vi "Radar-Vital-Sign.vi"() -> ()   [LabVIEW 2014]
doc: "Personal Daq 54 example.\nTriggering is immediate and readings are returned 1 scan at a time as available.\nBe sure to use the Acquisition Stop control for proper shutdown."
uses:
  <vilib>/Utility/error.llb/DialogType.ctl
  <vilib>/DAQmx/read.llb/DAQmx Read (Analog 1D DBL NChan 1Samp).vi
  <vilib>/Analysis/2dsp.llb/Complex FFT.vi
  <vilib>/DAQmx/create/channels.llb/DAQmx Create Channel (AI-Voltage-Basic).vi
  <vilib>/DAQmx/configure/timing.llb/DAQmx Timing (Sample Clock).vi
  <vilib>/DAQmx/miscellaneous.llb/DAQmx Fill In Error Info.vi
  <vilib>/measure/madcrms.llb/Basic Averaged DC-RMS for 1 Chan.vi
  Instance           2 26Saved   noise_Nov07_2009_5 .vi
  Instance          18 26Saved   noise_Nov07_2009_5 .vi
  Instance           4 26Saved   noise_Nov07_2009_5 .vi
  Instance           1 26Saved   noise_Nov07_2009_5 .vi
  <vilib>/measure/NI_MAPro.lvlib
  <vilib>/Analysis/NI_AALPro.lvlib
panel:
  in  "Save Data":bool
  in  "Max. Heartrate":i32=90
  in  "Min. Heartrate":i32=50
  out "Heartrate":dbl
  in  "Max. Resp. Rate":i32=30
  in  "Min. Resp. Rate":i32=10
  out "Resp. Rate":dbl
  in  "input terminal configuration":i32(ring)=10083 items=["default"=-1, "RSE"=10083, "NRSE"=10078, "Differential"=10106, "Pseudodifferential"=12529]
  in  "stop":bool
  in  "Maximum Value":dbl=5.0 format="%0.2f"
  in  "Minimum Value":dbl=-2.0 format="%0.2f"
  in  "Rate":dbl=20.0 caption="Sample Rate (Hz)" format="%0.2f"
  in  "Samples per Channel":i32=1
  out "Combined Spectrum":waveform(dbl)(graph)
  in  "FFT":i32=256
  out "I/Q Signal":dynamicdata(graph)
  in  "t0":timestamp=timestamp(3198752888.296 s since 1904-01-01)
  # "Radar Noncontact Vital Sign Detection\n\nby C.Gu, April 2012\n@ Texas Tech"
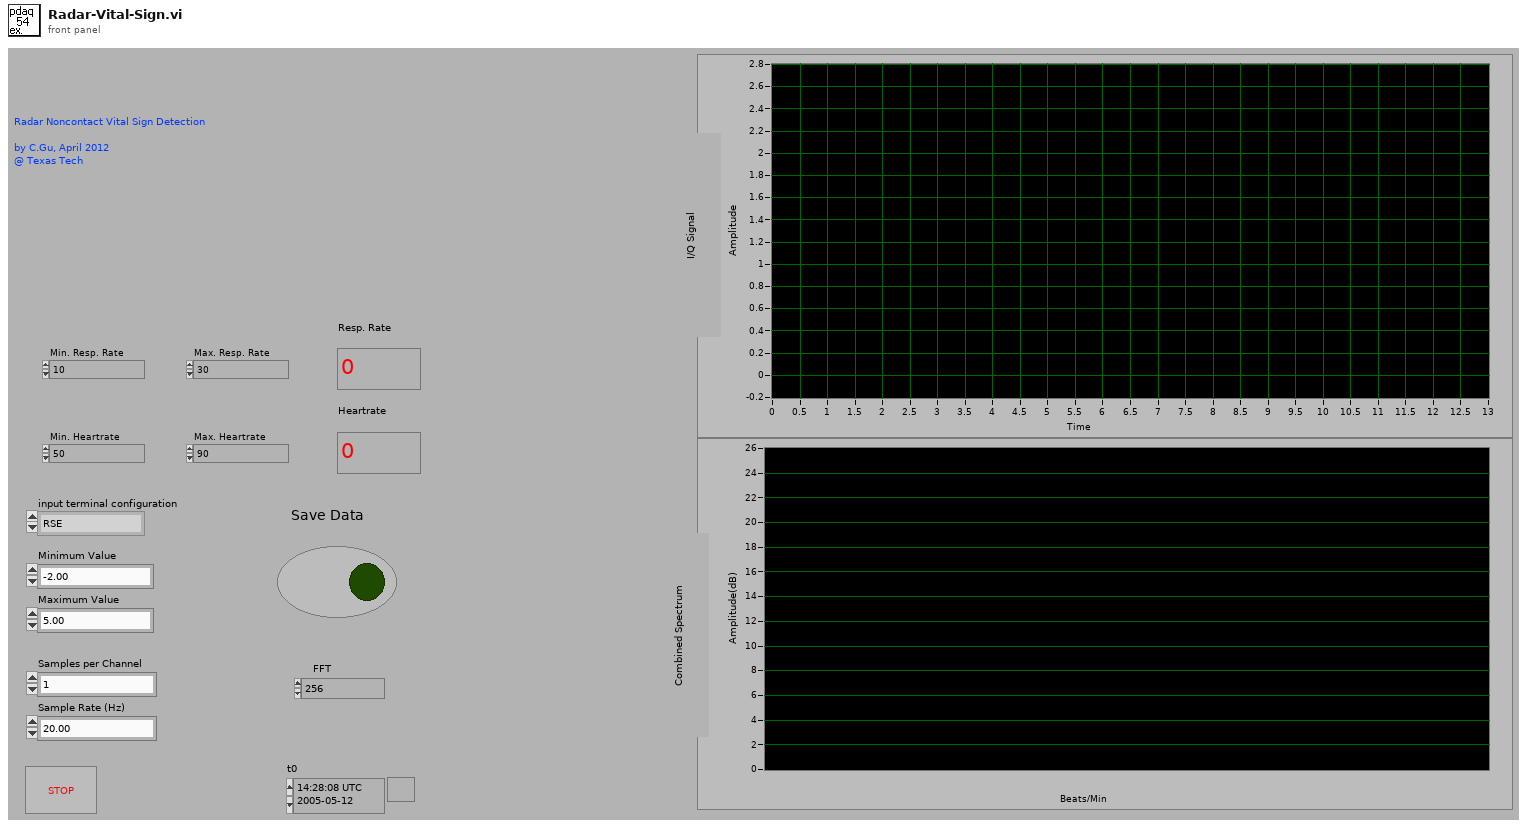
[diagram p1: front panel]
types:
  T1 = typedef "DialogType.ctl" = u16
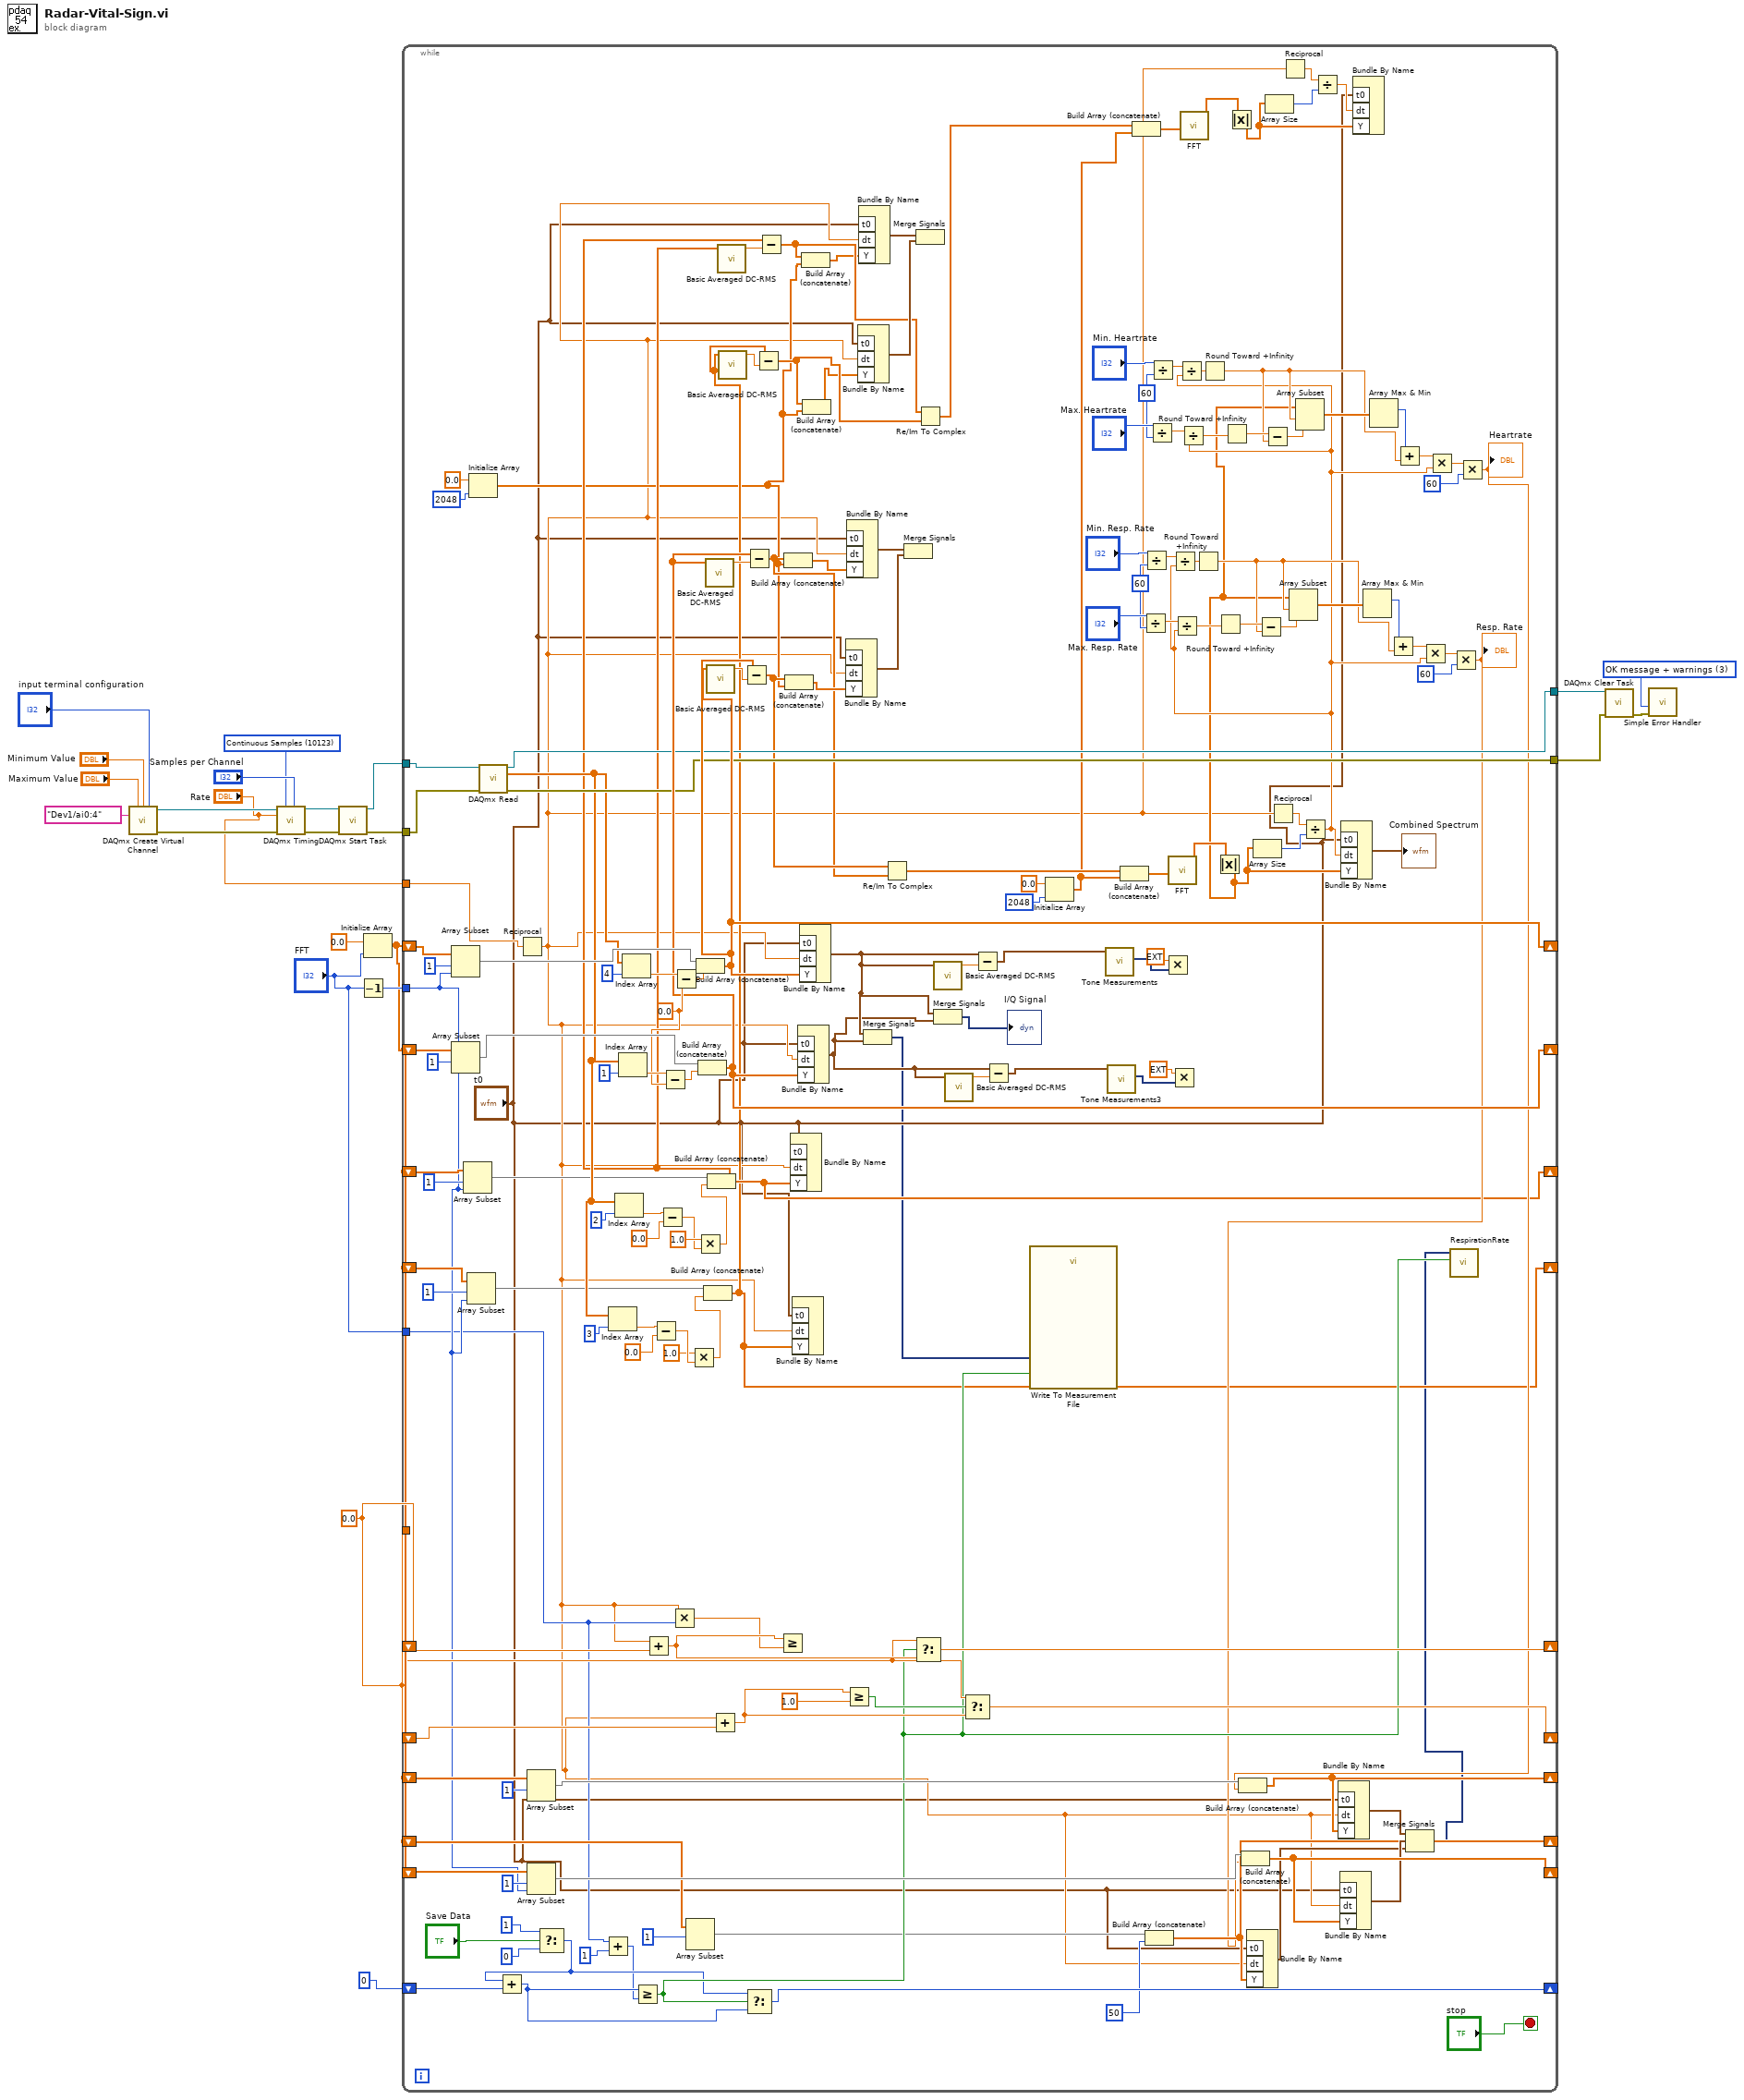
[diagram p0: block diagram]
diagram:
  w3 = 0.0 ("element")
  w9 = T1 3 items=["no dialog", "OK message", "continue or stop message", "OK message + warnings", "continue/stop + warnings"] ("type of dialog (OK msg:1)")
  w16 = 10123 items=["Finite Samples"=10178, "Continuous Samples"=10123] ("sample mode")
  n1 = call-poly <vilib>:"DAQmx Create Virtual Channel.vi"("maximum value"="Maximum Value", "minimum value"="Minimum Value", "input terminal configuration"="input terminal configuration", "physical channels"=tag "Dev1/ai0:4") -> ("task out"=w17:refnum<k21>, "error out"=w19:errorcluster)  [unwired: 5 in, 5 out]
  n2 = call-poly <vilib>:"DAQmx Timing.vi"("task/channels in"=w17, "sample mode"=w16, "samples per channel"="Samples per Channel", "rate"="Rate", "error in"=w19) -> ("task out"=w15:refnum<k21>, "error out"=w14:errorcluster)  [unwired: 2 in, 7 out]
  n3 = call <vilib>:"DAQmx Start Task.vi"("task/channels in"=w15, "error in"=w14) -> ("task out"=w12:refnum<k21>, "error out"=w11:errorcluster)  [unwired: 12 out]
  n4 = Decrement(x="FFT") -> (x-1=w22:i32)
  n5 = Initialize Array(0.0 ("element"), "FFT") -> (w1:dbl[])
  n6 = while {
    shift-right: [w156] -> _
    shift-left: w1 -> [w186]
    tunnel: w22 -> [w62]
    shift-right: [w155] -> _
    shift-left: w1 -> [w177]
    tunnel: w12 -> [w154]
    tunnel: w11 -> [w153]
    tunnel: "Rate" -> [w152]
    tunnel: [w151] -> w8
    tunnel: [w150] -> w7
    shift-right: [w145] -> _
    shift-left: w3 -> [w143]
    tunnel: "FFT" -> [w51]
    tunnel: w3 -> [w137]
    shift-right: [w141] -> _
    shift-left: w3 -> [w138]
    shift-right: [w125] -> _
    shift-left: w1 -> [w131]
    shift-right: [w126] -> _
    shift-left: w1 -> [w128]
    shift-right: [w86] -> _
    shift-left: 0 -> [w88]
    shift-right: [w44] -> _
    shift-left: w1 -> [w79]
    shift-right: [w70] -> _
    shift-left: w1 -> [w74]
    shift-right: [w43] -> _
    shift-left: w1 -> [w64]
    stop <- "stop" stop-if-true
    w91 = 60
    w106 = 60
    w171 = 0.0 ("element")
    n7 = Array Subset(array=w186, index=1, length=w62) -> (w184:dbl[])
    n8 = Array Subset(array=w177, index=1, length=w62) -> (w175:dbl[])
    n9 = Array Subset(array=w79, index=1, length=w62) -> (w45:dbl[])
    n10 = Array Subset(array=w64, index=1, length=w62) -> (w54:dbl[])
    n11 = Initialize Array(0.0 ("element"), 2048 ("dimension size")) -> (w40:dbl[])
    n12 = call-poly <vilib>:"DAQmx Read.vi"("task/channels in"=w154, "error in"=w153) -> ("task out"=w151:refnum<k21>, "data"=w55:dbl[], "error out"=w150:errorcluster)  [unwired: 11 out]
    n13 = Reciprocal(x=w152) -> (1/x=w29:dbl)
    n14 = Array Subset(array=w128, index=1) -> (w127:dbl[])  [unwired: 1 in]
    n15 = Array Subset(array=w131, index=1, length=w62) -> (w130:dbl[])
    n16 = Select(t=1, s="Save Data", f=0) -> (s? t:f=w82:i32)
    n17 = Add(x=w82, y=w88) -> (x+y=w87:i32)
    n18 = Add(x=w51, y=1 ("index")) -> (x+y=w50:i32)
    n19 = Index Array(array=w55, index=3 ("index (row)")) -> (element=w58:dbl)
    n20 = Index Array(array=w55, index=2 ("index (row)")) -> (element=w76:dbl)
    n21 = Index Array(array=w55, index=1 ("index (row)")) -> (element=w172:dbl)
    n22 = Index Array(array=w55, index=4 ("index (row)")) -> (element=w173:dbl)
    n23 = Greater Or Equal?(x=w87, y=w50) -> (x >= y?=w85:bool)
    n24 = Add(x=w29, y=w143) -> (x+y=w146:dbl)
    n25 = Subtract(x=w58, y=0.0 ("element")) -> (x-y=w61:dbl)
    n26 = Subtract(x=w76, y=0.0 ("element")) -> (x-y=w66:dbl)
    n27 = Subtract(x=w172, y=w171) -> (x-y=w165:dbl)
    n28 = Multiply(x=w29, y=w51) -> (x*y=w144:dbl)
    n29 = Subtract(x=w173, y=w171) -> (x-y=w166:dbl)
    n30 = Array Subset(array=w74, index=1) -> (w72:dbl[])  [unwired: 1 in]
    n31 = Multiply(x=1.0, y=w61) -> (x*y=w56:dbl)
    n32 = Build Array (concatenate)(w184, w166) -> (w156:dbl[])
    n33 = Multiply(x=1.0, y=w66) -> (x*y=w65:dbl)
    n34 = Build Array (concatenate)(w175, w165) -> (w155:dbl[])
    n35 = Build Array (concatenate)(w54, w56) -> (w43:dbl[])
    n36 = call-poly <vilib>:"Basic Averaged DC-RMS.vi"("signal in"=w155) -> ("DC value"=w164:dbl)  [unwired: 4 in, 6 out]
    n37 = call-poly <vilib>:"Basic Averaged DC-RMS.vi"("signal in"=w156) -> ("DC value"=w163:dbl)  [unwired: 4 in, 6 out]
    n38 = Build Array (concatenate)(w45, w65) -> (w44:dbl[])
    n39 = Add(x=w29, y=w138) -> (x+y=w142:dbl)
    n40 = call-poly <vilib>:"Basic Averaged DC-RMS.vi"("signal in"=w44) -> ("DC value"=w46:dbl)  [unwired: 4 in, 6 out]
    n41 = call-poly <vilib>:"Basic Averaged DC-RMS.vi"("signal in"=w43) -> ("DC value"=w47:dbl)  [unwired: 4 in, 6 out]
    n42 = Subtract(x=w156, y=w163) -> (x-y=w148:dbl[])
    n43 = Subtract(x=w155, y=w164) -> (x-y=w147:dbl[])
    n44 = Select(t=w82, s=w85, f=w87) -> (s? t:f=w86:i32)
    n45 = Subtract(x=w43, y=w47) -> (x-y=w42:dbl[])
    n46 = Subtract(x=w44, y=w46) -> (x-y=w39:dbl[])
    n47 = Greater Or Equal?(x=w146, y=w144) -> ()  [unwired: 1 out]
    n48 = Build Array (concatenate)(w147, w40) -> (w169:dbl[])
    n49 = Build Array (concatenate)(w148, w40) -> (w170:dbl[])
    n50 = Bundle By Name("t0"="t0", "dt"=w29, "Y"=w44) -> ()  [unwired: 2 out]
    n51 = Bundle By Name("t0"="t0", "dt"=w29, "Y"=w43) -> ()  [unwired: 2 out]
    n52 = Bundle By Name("t0"="t0", "dt"=w29, "Y"=w155) -> (w25:waveform(dbl))  [unwired: 1 out]
    n53 = Bundle By Name("t0"="t0", "dt"=w29, "Y"=w156) -> (w26:waveform(dbl))  [unwired: 1 out]
    n54 = Build Array (concatenate)(w39, w40) -> (w38:dbl[])
    n55 = Build Array (concatenate)(w42, w40) -> (w41:dbl[])
    n56 = Greater Or Equal?(x=w142, y=1.0) -> (x >= y?=w139:bool)
    n57 = Bundle By Name("t0"="t0", "dt"=w29, "Y"=w170) -> (w161:waveform(dbl))  [unwired: 1 out]
    n58 = Bundle By Name("t0"="t0", "dt"=w29, "Y"=w169) -> (w162:waveform(dbl))  [unwired: 1 out]
    n59 = Bundle By Name("t0"="t0", "dt"=w29, "Y"=w41) -> (w49:waveform(dbl))  [unwired: 1 out]
    n60 = Bundle By Name("t0"="t0", "dt"=w29, "Y"=w38) -> (w48:waveform(dbl))  [unwired: 1 out]
    n61 = Merge Signals(w26, w25) -> (w24:dynamicdata)
    n62 = Re/Im To Complex(1:w147, 2:w148) -> (0:w167:cdb[])
    n63 = Merge Signals(w162, w161) -> ()  [unwired: 1 out]
    n64 = Select(t=w137, s=w85, f=w146) -> (s? t:f=w145:dbl)
    n65 = Merge Signals(w48, w49) -> ()  [unwired: 1 out]
    n66 = Re/Im To Complex(1:w42, 2:w39) -> (0:w30:cdb[])
    n67 = call-poly <vilib>:"Basic Averaged DC-RMS.vi"("signal in"=w26) -> ("DC value"=w136:dbl)  [unwired: 4 in, 6 out]
    n68 = Merge Signals(w26, w25) -> (→"I/Q Signal":dynamicdata)
    n69 = call-poly <vilib>:"Basic Averaged DC-RMS.vi"("signal in"=w25) -> ("DC value"=w134:dbl)  [unwired: 4 in, 6 out]
    n70 = Select(t=w137, s=w139, f=w142) -> (s? t:f=w141:dbl)
    n71 = Subtract(x=w26, y=w136) -> (x-y=w135:waveform(dbl))
    n72 = Subtract(x=w25, y=w134) -> (x-y=w133:waveform(dbl))
    n73 = call "Write To Measurement File"("Signals"=w24, "Enable"=w85) -> ()  [unwired: 5 in, 13 out]
    n74 = Initialize Array(0.0 ("element"), 2048 ("dimension size")) -> (w31:dbl[])
    n75 = call "Tone Measurements"("Signals"=w135) -> ("Frequency"=w181:dynamicdata)  [unwired: 1 in, 9 out]
    n76 = call "Tone Measurements3"("Signals"=w133) -> ("Frequency"=w178:dynamicdata)  [unwired: 1 in, 9 out]
    n77 = Build Array (concatenate)(w167, w31) -> (w157:cdb[])
    n78 = Build Array (concatenate)(w30, w31) -> (w34:cdb[])
    n79 = Divide(x="Max. Resp. Rate", y=w106) -> (x/y=w120:dbl)
    n80 = Divide(x="Min. Resp. Rate", y=w106) -> (x/y=w121:dbl)
    n81 = Build Array (concatenate)(w72, 50 ("index")) -> (w70:dbl[])
    n82 = Divide(x="Max. Heartrate", y=w91) -> (x/y=w104:dbl)
    n83 = Divide(x="Min. Heartrate", y=w91) -> (x/y=w105:dbl)
    n84 = Multiply(x=ext 60.0, y=w181) -> ()  [unwired: 1 out]
    n85 = call-poly <vilib>:"FFT.vi"("X"=w157) -> ("FFT {X}"=w160:cdb[])  [unwired: 2 in, 8 out]
    n86 = Multiply(x=ext 60.0, y=w178) -> ()  [unwired: 1 out]
    n87 = call-poly <vilib>:"FFT.vi"("X"=w34) -> ("FFT {X}"=w32:cdb[])  [unwired: 2 in, 8 out]
    n88 = Absolute Value(x=w160) -> (abs(x)=w80:dbl[])
    n89 = Absolute Value(x=w32) -> (abs(x)=w37:dbl[])
    n90 = Bundle By Name("t0"="t0", "dt"=w29, "Y"=w70) -> (w71:waveform(dbl))  [unwired: 1 out]
    n91 = Array Size(array=w80) -> (size(s)=w158:i32)
    n92 = Array Size(array=w37) -> (size(s)=w33:i32)
    n93 = Reciprocal(x=w29) -> (1/x=w109:dbl)
    n94 = Reciprocal(x=w29) -> (1/x=w35:dbl)
    n95 = Divide(x=w109, y=w158) -> (x/y=w90:dbl)
    n96 = Divide(x=w121, y=w90) -> (x/y=w119:dbl)
    n97 = Divide(x=w120, y=w90) -> (x/y=w118:dbl)
    n98 = Divide(x=w105, y=w90) -> (x/y=w103:dbl)
    n99 = Divide(x=w104, y=w90) -> (x/y=w102:dbl)
    n100 = Round Toward +Infinity(x=w119) -> (ceil(x): smallest int >= x=w113:dbl)
    n101 = Round Toward +Infinity(x=w103) -> (ceil(x): smallest int >= x=w97:dbl)
    n102 = Round Toward +Infinity(x=w118) -> (ceil(x): smallest int >= x=w116:dbl)
    n103 = Round Toward +Infinity(x=w102) -> (ceil(x): smallest int >= x=w100:dbl)
    n104 = Subtract(x=w116, y=w113) -> (x-y=w117:dbl)
    n105 = Subtract(x=w100, y=w97) -> (x-y=w101:dbl)
    n106 = Array Subset(array=w80, index=w113, length=w117) -> (w115:dbl[])
    n107 = Array Subset(array=w80, index=w97, length=w101) -> (w99:dbl[])
    n108 = Divide(x=w35, y=w33) -> (x/y=w36:dbl)
    n109 = Bundle By Name("t0"="t0", "dt"=w90, "Y"=w80) -> (→"Combined Spectrum":waveform(dbl))  [unwired: 1 out]
    n110 = Bundle By Name("t0"="t0", "dt"=w36, "Y"=w37) -> ()  [unwired: 2 out]
    n111 = Array Max & Min(array=w115) -> (max index (indices)=w114:i32)  [unwired: 3 out]
    n112 = Array Max & Min(array=w99) -> (max index (indices)=w98:i32)  [unwired: 3 out]
    n113 = Add(x=w114, y=w113) -> (x+y=w112:dbl)
    n114 = Add(x=w98, y=w97) -> (x+y=w96:dbl)
    n115 = Multiply(x=w112, y=w90) -> (x*y=w111:dbl)
    n116 = Multiply(x=w96, y=w90) -> (x*y=w95:dbl)
    n117 = Multiply(x=w111, y=60) -> (x*y=w69:dbl)
    "Resp. Rate" <- w69
    n118 = Build Array (concatenate)(w130, w69) -> (w125:dbl[])
    n119 = Bundle By Name("t0"="t0", "dt"=w29, "Y"=w125) -> (w123:waveform(dbl))  [unwired: 1 out]
    n120 = Multiply(x=w95, y=60) -> (x*y=w89:dbl)
    "Heartrate" <- w89
    n121 = Build Array (concatenate)(w127, w89) -> (w126:dbl[])
    n122 = Bundle By Name("t0"="t0", "dt"=w29, "Y"=w126) -> (w124:waveform(dbl))  [unwired: 1 out]
    n123 = Merge Signals(w124, w123, w71) -> (w27:dynamicdata)
    n124 = call "RespirationRate"("Enable"=w85, "Signals"=w27) -> ()  [unwired: 3 in, 7 out]
  }
  n125 = call <vilib>:"DAQmx Clear Task.vi"("task in"=w8, "error in"=w7) -> ("error out"=w6:errorcluster)  [unwired: 13 out]
  n126 = call <vilib>:"Simple Error Handler.vi"("type of dialog (OK msg:1)"=w9, "error in (no error)"=w6) -> ()  [unwired: 8 out]
